vi "Results_Get_ReadFast.vi"(11 "Results":dbl[](array[numeric])) -> (1 "Position":dbl[](array[numeric]), 2 "Velocity":dbl)   [LabVIEW 2017, in "WordManipulationLibrary.lvlib"]
uses:
  WordManipulationLibrary.lvlib
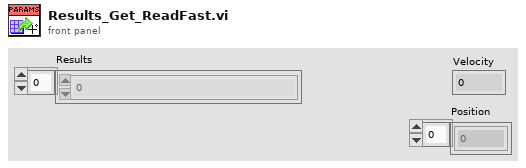
[diagram p1: front panel]
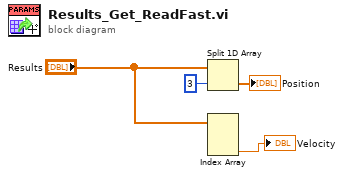
[diagram p0: block diagram]
diagram:
  n1 = Split 1D Array(array="Results", index=3) -> (second subarray=→"Position":dbl[])  [unwired: 1 out]
  n2 = Index Array(array="Results") -> (element #3=→"Velocity":dbl)  [unwired: 3 in, 2 out]
